vi "Ouptut_Sound_trace_nm.vi"() -> (5 "Plug in titles":string[](array[string]), 7 "Plug in values":string[](array[string]))   [LabVIEW 2010]
doc: "This VI demonstrates how to output continuous sound using SO Set Num Buffers. This example is available only on Windows."
uses:
  <vilib>/sound2/lvsound2.llb/Sound Data Format.ctl
  <vilib>/sound2/lvsound2.llb/Sampling Mode.ctl
  Globals/Meas_global.vi
  <vilib>/sound2/lvsound2.llb/Sound Output Write (DBL Single).vi
  <vilib>/measure/NI_MABase.lvlib
panel:
  out "trace length":dbl
  in  "A delta":dbl=0.1
  in  "Start A":dbl=0.7
  in  "End A":dbl=1.0
  out "Desired Amplitudes":dbl[](array[numeric])=[40.0, 80.0, 120.0, 160.0, 200.0, 240.0, 280.0, 320.0, 360.0, 400.0, 440.0, 480.0, 520.0, 560.0, 600.0, 640.0, 680.0, 720.0, 760.0, 800.0, 840.0, 880.0, 920.0, 960.0, 1000.0, 1040.0, 1080.0, 1120.0, 1160.0, 1200.0, 1240.0, 1280.0, 1320.0, 1360.0, 1400.0, 1440.0, 1480.0, 1520.0, 1560.0, 1600.0]
  in  "Device ID 2":u32
  in  "F delta":dbl=100.0
  in  "Start F":dbl=1000.0
  in  "End F":dbl=2000.0
  out "Desired Frequencies":dbl[](array[numeric])=[40.0, 80.0, 120.0, 160.0, 200.0, 240.0, 280.0, 320.0, 360.0, 400.0, 440.0, 480.0, 520.0, 560.0, 600.0, 640.0, 680.0, 720.0, 760.0, 800.0, 840.0, 880.0, 920.0, 960.0, 1000.0, 1040.0, 1080.0, 1120.0, 1160.0, 1200.0, 1240.0, 1280.0, 1320.0, 1360.0, 1400.0, 1440.0, 1480.0, 1520.0, 1560.0, 1600.0]
  in  "Dwell Time (s)":dbl=0.1
  in  "Number of Cycles":i32=30
  in  "Sound Format":T1={"sample rate (S/s)"=96000.0, "number of channels"=1, "bits per sample"=24}
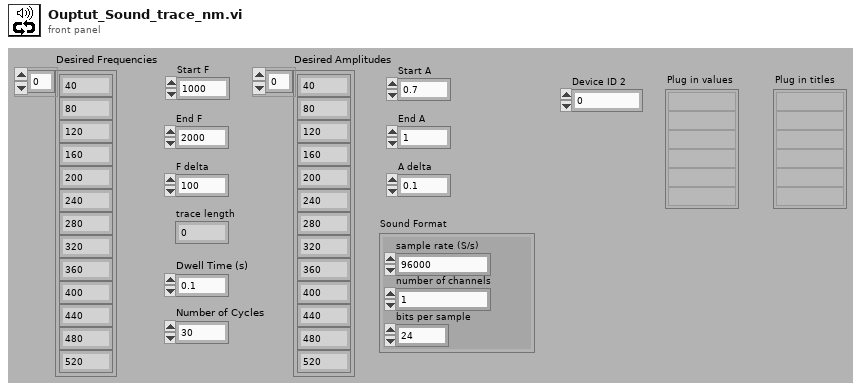
[diagram p1: front panel]
types:
  T1 = typedef "Sound Data Format.ctl" = cluster{"sample rate (S/s)":dbl, "number of channels":i32, "bits per sample":i32}
  T2 = typedef "Post_Process.ctl" = enum16{"Take New Data", "Post Process Raw Data File"}
  T3 = typedef "Sampling Mode.ctl" = i32
  T4 = typedef "Sound Output Task ID.ctl" = u32
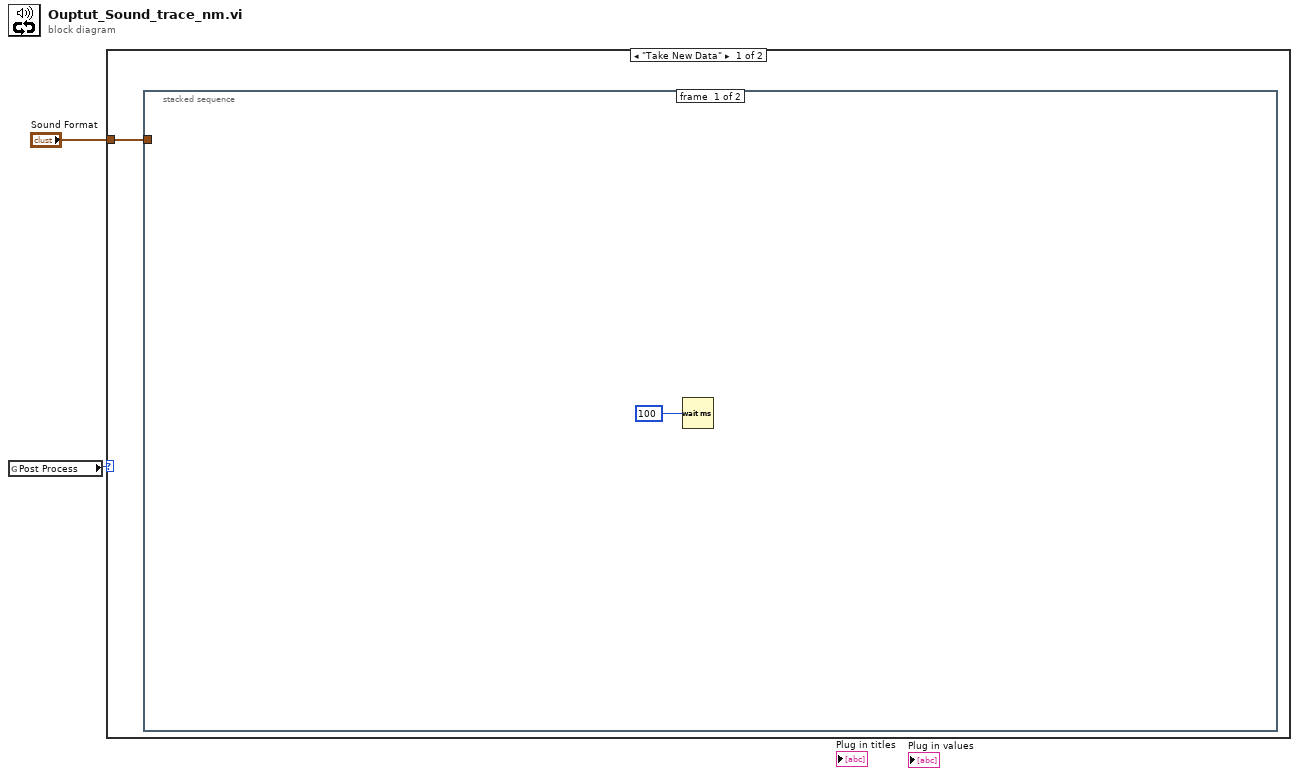
[diagram p0: block diagram]
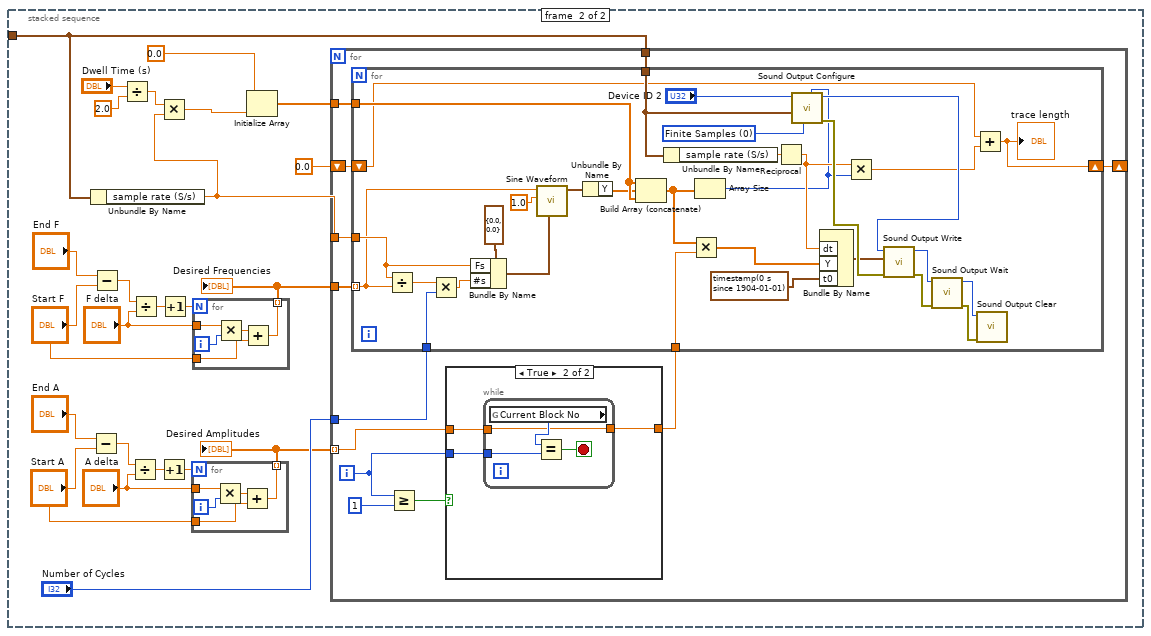
[diagram p2: hidden frame]
diagram:
  n1 = global read "Meas_global.vi" "Post Process"() -> (w2:T2)
  n2 = case shown="\"Take New Data\"" w2 {
    tunnel: "Sound Format" -> [w3 _]
    frame "Take New Data" {
      n3 = stacked-sequence {
        tunnel: w3 -> [_ w13]
        frame #0 {
          n4 = Wait (ms)(milliseconds to wait=u32 100) -> ()  [unwired: 1 out]
        }
        frame #1 {
          n5 = Unbundle By Name(w13) -> ("sample rate (S/s)"=w27:dbl)
          n6 = Subtract(x="End A", y="Start A") -> (x-y=w7:dbl)
          n7 = Subtract(x="End F", y="Start F") -> (x-y=w17:dbl)
          n8 = Divide(x="Dwell Time (s)", y=2.0) -> (x/y=w16:dbl)
          n9 = Divide(x=w7, y="A delta") -> (x/y=w9:dbl)
          n10 = Divide(x=w17, y="F delta") -> (x/y=w19:dbl)
          n11 = Multiply(x=w16, y=w27) -> (x*y=w25:dbl)
          n12 = Increment(x=w9) -> (x+1=w10:dbl)
          n13 = Increment(x=w19) -> (x+1=w20:dbl)
          n14 = for {
            N: w10 -> [_]
            tunnel: [w31] -> w6 mode=indexing
            tunnel: "Start A" -> [w30]
            tunnel: "A delta" -> [w29]
            i -> [w33]
            n15 = Multiply(x=w29, y=w33) -> (x*y=w32:dbl)
            n16 = Add(x=w32, y=w30) -> (x+y=w31:dbl)
          }
          "Desired Amplitudes" <- w6
          n17 = for {
            N: w20 -> [_]
            tunnel: [w36] -> w14 mode=indexing
            tunnel: "Start F" -> [w35]
            tunnel: "F delta" -> [w34]
            i -> [w38]
            n18 = Multiply(x=w34, y=w38) -> (x*y=w37:dbl)
            n19 = Add(x=w37, y=w35) -> (x+y=w36:dbl)
          }
          "Desired Frequencies" <- w14
          n20 = Initialize Array(0.0 ("element"), w25) -> (w23:dbl[])
          n21 = for {
            tunnel: w27 -> [w50]
            tunnel: w14 -> [w48]
            tunnel: "Number of Cycles" -> [w49]
            tunnel: w23 -> [w47]
            tunnel: w6 -> [w42] mode=indexing
            tunnel: w13 -> [w46]
            shift-right: [w44] -> _
            shift-left: 0.0 -> [w45]
            i -> [w39]
            n22 = Greater Or Equal?(x=w39, y=1) -> (x >= y?=w40:bool)
            n23 = case shown="True" w40 {
              tunnel: w39 -> [_ w54]
              tunnel: [w51 w53] -> w43
              tunnel: w42 -> [w51 w52]
              frame False {
              }
              frame True {
                n24 = while {
                  tunnel: w54 -> [w58]
                  tunnel: [w55] -> w53
                  tunnel: w52 -> [w55]
                  stop <- w56 stop-if-true
                  n25 = global read "Meas_global.vi" "Current Block No"() -> (w57:i32)
                  n26 = Equal?(x=w57, y=w58) -> (x = y?=w56:bool)
                }
              }
            }
            n27 = for {
              tunnel: w50 -> [w88]
              tunnel: w49 -> [w87]
              tunnel: w48 -> [w82] mode=indexing
              tunnel: w47 -> [w81]
              tunnel: w46 -> [w75]
              shift-right: [w64] -> w44
              shift-left: w45 -> [w66]
              tunnel: w43 -> [w59]
              w76 = T3 0 items=["Finite Samples", "Continuous Samples"] ("sample mode")
              n28 = Divide(x=w88, y=w82) -> (x/y=w85:dbl)
              n29 = Multiply(x=w85, y=w87) -> (x*y=w86:dbl)
              n30 = Bundle By Name(cluster=cluster{"Fs":dbl, "#s":dbl} {"Fs"=0.0, "#s"=0.0} ("sampling info"), "Fs"=w88, "#s"=w86) -> (w84:cluster{"Fs":dbl, "#s":dbl})
              n31 = call <vilib>:"Sine Waveform.vi"("sampling info"=w84, "amplitude"=1.0, "frequency"=w82) -> ("signal out"=w83:waveform(dbl))  [unwired: 7 in, 1 out]
              n32 = Unbundle By Name(w83) -> ("Y"=w80:dbl[])
              n33 = Build Array (concatenate)(w81, w80, w81) -> (w63:dbl[])
              n34 = Unbundle By Name(w75) -> ("sample rate (S/s)"=w78:dbl)
              n35 = Multiply(x=w63, y=w59) -> (x*y=w62:dbl[])
              n36 = Array Size(array=w63) -> (size(s)=w67:i32)
              n37 = Reciprocal(x=w78) -> (1/x=w68:dbl)
              n38 = call <vilib>:"Sound Output Configure.vi"("number of samples/ch"=w67, "sample mode"=w76, "sound format"=w75, "device ID"="Device ID 2") -> ("error out"=w74:errorcluster, "task ID"=w73:T4)  [unwired: 6 in]
              n39 = Bundle By Name("dt"=w68, "Y"=w62, "t0"=timestamp(0 s since 1904-01-01)) -> (w60:waveform(dbl))  [unwired: 1 out]
              n40 = Multiply(x=w68, y=w67) -> (x*y=w65:dbl)
              n41 = call-poly <vilib>:"Sound Output Write.vi"("error in (no error)"=w74, "data"=w60, "task ID"=w73) -> ("error out"=w70:errorcluster, "task ID out"=w72:T4)  [unwired: 7 in]
              n42 = call <vilib>:"Sound Output Wait.vi"("error in (no error)"=w70, "task ID"=w72) -> ("error out"=w69:errorcluster, "task ID out"=w71:T4)  [unwired: 8 in]
              n43 = Add(x=w66, y=w65) -> (x+y=w64:dbl)
              "trace length" <- w64
              n44 = call <vilib>:"Sound Output Clear.vi"("error in (no error)"=w69, "task ID"=w71) -> ()  [unwired: 9 in, 1 out]
            }
          }
        }
      }
    }
    frame "Post Process Raw Data File" {
    }
  }
